vi "Size.vi"(8 "error in (no error)":errorcluster, 11 "MessageQ in":refnum<class "MessageQ.lvclass">) -> (0 "error out":errorcluster, 1 "Max Size":i32, 2 "Depth":i32, 3 "MessageQ out":refnum<class "MessageQ.lvclass">)   [LabVIEW 2020, in "Volatus.lvlib" / "MessageQ.lvclass"]
uses:
  MessageQ.lvclass
  MessageQ.lvclass/MessageQ.ctl
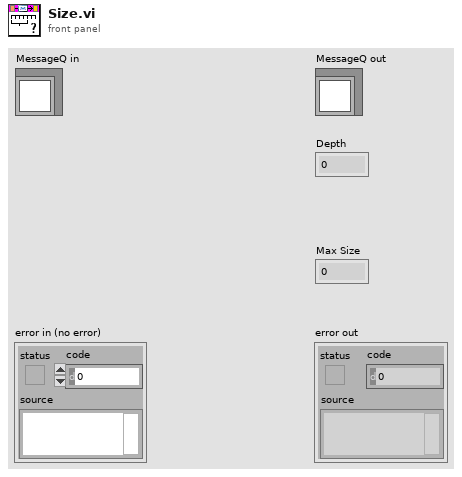
[diagram p1: front panel]
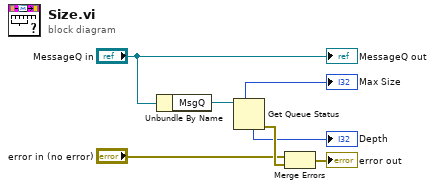
[diagram p0: block diagram]
diagram:
  n1 = Unbundle By Name("MessageQ in") -> ("MsgQ"=w4:refnum<queue>)
  n2 = Get Queue Status(queue=w4) -> (max queue size=→"Max Size":i32, error out=w7:errorcluster, # elements in queue=→"Depth":i32)  [unwired: 2 in, 5 out]
  n3 = Merge Errors("error in (no error)", w7) -> (→"error out":errorcluster)
  "MessageQ out" <- "MessageQ in"
